vi "dataset.name.vi"(8 "error in":errorcluster, 11 "Dataset in":refnum<class "Dataset.lvclass">) -> (0 "error out":errorcluster, 3 "Dataset out":refnum<class "Dataset.lvclass">)   [LabVIEW 2020, in "Dataset.lvclass"]
doc: "Returns the dataset's name."
uses:
  Dataset.lvclass
  Dataset.lvclass/Dataset.ctl
  client.lvlib
panel:
  out "out_needed out":u32
  out "name":string
  in  "buf":string
  in  "cap":u32
  in  "out_needed":u32
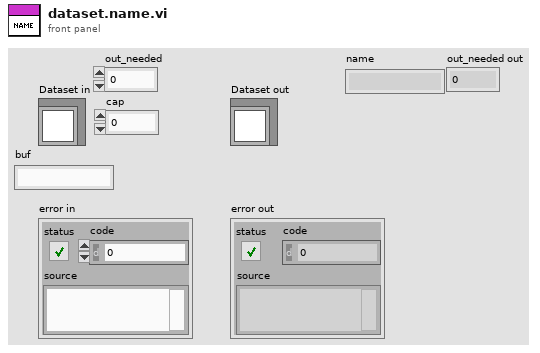
[diagram p1: front panel]
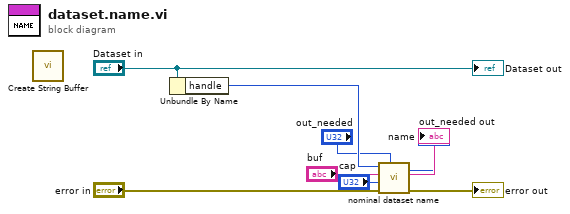
[diagram p0: block diagram]
diagram:
  n1 = call "Create String Buffer.vi"() -> ()  [unwired: 9 in, 3 out]
  n2 = Unbundle By Name("Dataset in") -> ("handle"=w7:i32)
  n3 = call "nominal dataset name.vi"("out_needed"="out_needed", "error in (no error)"="error in", "cap"="cap", "buf"="buf", "dataset"=w7) -> ("error out"=→"error out":errorcluster, "buf out"=→"name":string, "out_needed out"=→"out_needed out":u32)  [unwired: 3 in, 1 out]
  "Dataset out" <- "Dataset in"
